vi "To and From CSV.vi"() -> (0 "error out":errorcluster, 3 "Pass":bool)   [LabVIEW 2014, in "Scan Engine tests.lvlib"]
uses:
  Scan Engine tests.lvlib
  <vilib>/NI/Module Execution Interface/Engine Configuration/engine configuration.lvclass
  editor node/Scan Engine editor node.lvclass
  <vilib>/NI/Configuration Framework/serializable configuration/NISE_CEF_serializable configuration.lvclass/NISE_CEF_serializable configuration.ctl
  configuration/Scan Engine configuration.lvclass/Scan Engine configuration.ctl
  <vilib>/Utility/LVClass/Get LV Class Name.vi
  <vilib>/NI/Configuration Framework/error generator/NISE_error generator.vi
  <vilib>/NI/Tag Bus Module Framework/channel/TBM channel.lvclass
  <vilib>/NI/Configuration Framework/serializable configuration/NISE_CEF_serializable configuration.lvclass
  configuration/Scan Engine configuration.lvclass
panel:
  out "Object":bool
  out "Lines":bool
  out "Write Channels":bool
  out "Read Channels":bool
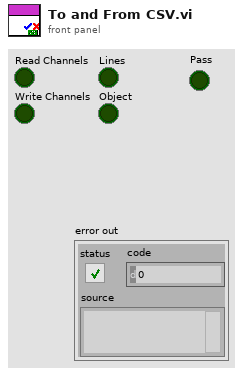
[diagram p1: front panel]
types:
  T1 = typedef "Scan Engine configuration.lvclass/Line.ctl" = cluster{"channel":refnum<class "TBM channel.lvclass">, "Tag":string}
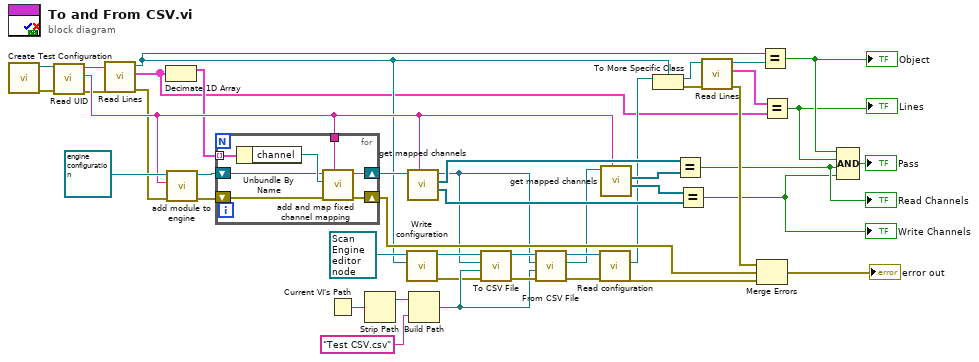
[diagram p0: block diagram]
diagram:
  n1 = call "Create Test Configuration.vi"() -> ("error out"=w3:errorcluster, "module"=w44:refnum<class "Scan Engine configuration.lvclass">)  [unwired: 6 in, 4 out]
  n2 = call <vilib>:"Read UID.vi"("error in"=w3, "configuration in"=w44) -> ("error out"=w2:errorcluster, "instance id"=w34:string, "configuration out"=w43:refnum<class "Scan Engine configuration.lvclass">)  [unwired: 7 in]
  n3 = call "Read Lines.vi"("error in (no error)"=w2, "Scan Engine configuration in"=w43) -> ("error out"=w1:errorcluster, "Lines"=w6:T1[], "Scan Engine configuration out"=w9:refnum<class "Scan Engine configuration.lvclass">)  [unwired: 7 in]
  n4 = Decimate 1D Array(w6) -> (w33:T1[])  [unwired: 1 out]
  n5 = call-dynamic "add module to engine.vi"("error in"=w1, "module ID"=w34, "engine configuration in"=refnum<class "engine configuration.lvclass"> refnum ("engine configuration")) -> ("error out"=w35:errorcluster, "engine configuration out"=w41:refnum<class "engine configuration.lvclass">)  [unwired: 7 in]
  n6 = for {
    tunnel: w33 -> [w51] mode=indexing
    shift-right: [w49] -> w40
    shift-left: w41 -> [w48]
    tunnel: w34 -> [w47]
    shift-right: [w45] -> w19
    shift-left: w35 -> [w46]
    n7 = Unbundle By Name(w51) -> ("channel"=w50:refnum<class "TBM channel.lvclass">)
    n8 = call <vilib>:"add and map fixed channel mapping.vi"("module instance"=w47, "error in"=w46, "fixed channel"=w50, "engine configuration in"=w48) -> ("error out"=w45:errorcluster, "engine configuration out"=w49:refnum<class "engine configuration.lvclass">)  [unwired: 6 in]
  }
  n9 = Current VI's Path() -> (path=w25:path)
  n10 = Strip Path(path=w25) -> (stripped path=w24:path)  [unwired: 1 out]
  n11 = call-dynamic "Write configuration.vi"("configuration"=w9, "Scan Engine editor node in"=refnum<class "Scan Engine editor node.lvclass"> refnum ("Scan Engine editor node")) -> ("error out"=w21:errorcluster, "Scan Engine editor node out"=w30:refnum<class "Scan Engine editor node.lvclass">)  [unwired: 8 in]
  n12 = call-dynamic "get mapped channels.vi"("owner"=w34, "engine configuration in"=w40) -> ("write channels"=w36:refnum<class "TBM channel.lvclass">[], "read channels"=w39:refnum<class "TBM channel.lvclass">[], "engine configuration out"=w18:refnum<class "engine configuration.lvclass">)  [unwired: 5 in, 2 out]
  n13 = Build Path(base path=w24, name or relative path="Test CSV.csv") -> (appended path=w26:path)
  n14 = call-dynamic "To CSV File.vi"("error in (no error)"=w21, "Path"=w26, "engine configuration"=w18, "Scan Engine editor node in"=w30) -> ("error out"=w32:errorcluster, "Scan Engine editor node out"=w31:refnum<class "Scan Engine editor node.lvclass">)  [unwired: 6 in]
  n15 = call-dynamic "From CSV File.vi"("error in (no error)"=w32, "Path"=w26, "engine in"=w18, "Scan Engine editor node in"=w31) -> ("error out"=w29:errorcluster, "engine out"=w17:refnum<class "engine configuration.lvclass">, "Scan Engine editor node out"=w28:refnum<class "Scan Engine editor node.lvclass">)  [unwired: 4 in, 1 out]
  n16 = call-dynamic "Read configuration.vi"("error in"=w29, "Scan Engine editor node in"=w28) -> ("error out"=w23:errorcluster, "configuration"=w16:refnum<class "NISE_CEF_serializable configuration.lvclass">)  [unwired: 7 in, 1 out]
  n17 = call-dynamic "get mapped channels.vi"("owner"=w34, "engine configuration in"=w17) -> ("write channels"=w37:refnum<class "TBM channel.lvclass">[], "read channels"=w38:refnum<class "TBM channel.lvclass">[])  [unwired: 5 in, 3 out]
  n18 = To More Specific Class(target class=w9, reference=w16) -> (specific class reference=w14:refnum<class "Scan Engine configuration.lvclass">, error out=w15:errorcluster)  [unwired: 1 in]
  n19 = Equal?(x=w39, y=w38) -> (x = y?=w5:bool)
  "Read Channels" <- w5
  n20 = Equal?(x=w37, y=w36) -> (x = y?=w4:bool)
  "Write Channels" <- w4
  n21 = call "Read Lines.vi"("error in (no error)"=w15, "Scan Engine configuration in"=w14) -> ("error out"=w13:errorcluster, "Lines"=w7:T1[], "Scan Engine configuration out"=w8:refnum<class "Scan Engine configuration.lvclass">)  [unwired: 7 in]
  n22 = Merge Errors(w13, w19, w23) -> (→"error out":errorcluster)
  n23 = Equal?(x=w9, y=w8) -> (x = y?=w12:bool)
  "Object" <- w12
  n24 = Equal?(x=w7, y=w6) -> (x = y?=w11:bool)
  "Lines" <- w11
  n25 = Compound Arithmetic op=AND(w12, w11, w5, w4) -> (→"Pass":bool)
